vi "Unlock Data.vi"(8 "error in (no error)":errorcluster, 9 "Datum Type":variant, 10 "Datum Name":string, 11 "IModel in":refnum<class "IModel.lvclass">) -> (0 "error out":errorcluster, 3 "IModel out":refnum<class "IModel.lvclass">)   [LabVIEW 2020, in "MVA Framework.lvlib" / "IModel.lvlib" / "IModel.lvclass"]
doc: "解锁数据"
uses:
  IModel.lvclass
  IObserver/IObserver/IObserver.lvclass/IObserver.ctl
  IModel.lvclass/IModel.ctl
  IMediator/IMediator Messages/Unlock Publication Msg/Unlock Publication Msg.lvclass/Unlock Publication Msg.ctl
  composed-af-messages/Source/RoundTripMessage/RoundTripMessage.lvclass/RoundTripMessage.ctl
  <vilib>/ActorFramework/Message Enqueuer/Message Enqueuer.lvclass/Message Enqueuer.ctl
  composed-af-messages/Source/RoundTripMessage/Return Round-Trip Message.vi
  <vilib>/ActorFramework/Message Enqueuer/Enqueue.vi
  IMediator/IMediator Messages/Unlock Publication Msg/Unlock Publication Msg.lvclass
  composed-af-messages/Source/RoundTripMessage/RoundTripMessage.lvclass
  C:/Program Files/National Instruments/LabVIEW 2020/vi.lib/ActorFramework/Message/Message.lvclass
  <vilib>/ActorFramework/Message Priority Queue/Priority Enqueue.vi
  IObserver/IObserver/IObserver.lvclass
  C:/Program Files/National Instruments/LabVIEW 2020/vi.lib/ActorFramework/Actor/Actor.lvclass
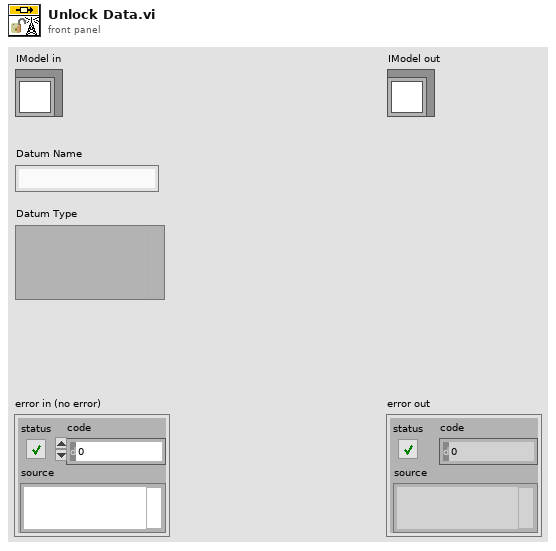
[diagram p1: front panel]
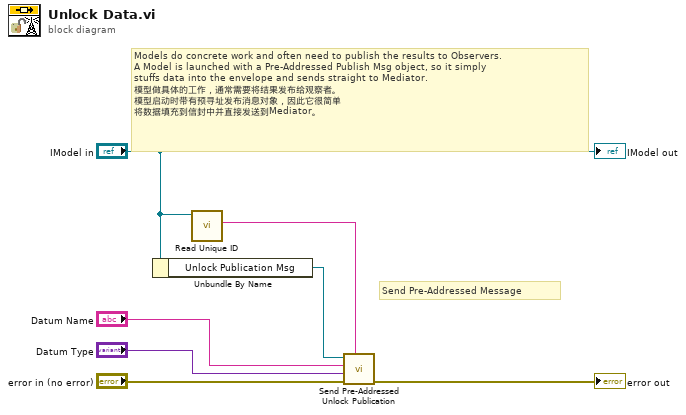
[diagram p0: block diagram]
diagram:
  # "Models do concrete work and often need to publish the results to Observers.\nA Model is launched with a Pre-Addressed Publish Msg object, so it simply\nstuffs data into the envelope and sends straight to Mediator.\n模型做具体的工作，通常需要将结果发布给观察者。\n模型启动时带有预寻址发布消息对象，因此它很简单\n将数据填充到信封中并直接发送到Mediator。"
  # "Send Pre-Addressed Message"
  n1 = Unbundle By Name("IModel in") -> ("Unlock Publication Msg"=w7:refnum<class "Unlock Publication Msg.lvclass">)
  n2 = call "Read Unique ID.vi"("IObserver In"="IModel in") -> ("Unique ID"=w1:string)  [unwired: 10 in]
  n3 = call "Send Pre-Addressed Unlock Publication.vi"("Publisher ID"=w1, "error in (no error)"="error in (no error)", "Data to Publish"="Datum Type", "Datum Name"="Datum Name", "Unlock Publication Msg"=w7) -> ("error out"=→"error out":errorcluster)  [unwired: 6 in]
  "IModel out" <- "IModel in"
